vi "LC1_Comm_main.vi"() -> ()   [LabVIEW 2016]
uses:
  <vilib>/DNP3/DNP3_Master/Operation Mode.ctl
  <vilib>/DNP3/DNP3_Master/Poll Binary Input Variation.ctl
  <vilib>/DNP3/DNP3_Master/Analog Variation.ctl
  <vilib>/DNP3/DNP3_Master/Poll Analog Input Variation.ctl
  <vilib>/DNP3/DNP3_Master/Response Type.ctl
  <vilib>/DNP3/DNP3_Master/Start Stop.ctl
  <vilib>/DNP3/DNP3_Master/Analog Info.ctl
  BESS_LC/LC_BESS_global.vi
  Communication/Global communication.vi
  Communication/Global communication output.vi
  Communication/DNP3 communication files/MGCC Communication Files/DNP3_Master_Station_MGCC.lvlib
  <vilib>/DNP3/DNP3_Master.lvlib
panel:
  out "Startup time":dbl
  out "Array":T3(array[cluster])=[{"DNP3 channel"="Master/Channel 160.36.56.202: 18000", "DNP3 master"="Master", "DNP3 master session"="Master/Channel 160.36.56.202: 18000/Master Session 7-8", "DNP3 command"="Master/Channel 160.36.56.202: 18000/Master Session 7-8/Command ", "MS_Network_Settings_Initial"={"Outstation IP"="160.36.56.202", "DNP3 Port"=18000, "DNP3 Master Address"=7, "DNP3 Outstation Address"=8}, "Ping status"=enum."Success", "PollD"=[{"start"=0, "stop"=5}], "PollA"=[{"start"=0, "stop"=5}], "error out"={"status"=FALSE, "code"=5103, "source"="DNP3_Master_Station_MGCC.lvlib:LC1_MS_Main.vi:580001<ERR>\nCommunication timeout\n\n\n<b>Complete call chain:</b>\n     DNP3_Master_Station_MGCC.lvlib:LC1_MS_Main.vi:580001\n     LC1_Comm_main.vi"}, "MS_RESET_IND"=FALSE}, {"DNP3 channel"="Master #1/Channel 160.36.56.201: 18000", "DNP3 master"="Master #1", "DNP3 master session"="Master #1/Channel 160.36.56.201: 18000/Master Session 5-6", "DNP3 command"="Master #1/Channel 160.36.56.201: 18000/Master Session 5-6/Command ", "MS_Network_Settings_Initial"={"Outstation IP"="160.36.56.201", "DNP3 Port"=18000, "DNP3 Master Address"=5, "DNP3 Outstation Address"=6}, "Ping status"=enum."Success", "PollD"=[{"start"=0, "stop"=5}], "PollA"=[{"start"=0, "stop"=5}], "error out"={"status"=FALSE, "code"=5103, "source"="DNP3_Master_Station_MGCC.lvlib:LC1_MS_Main.vi:580001<ERR>\nCommunication timeout\n\n\n<b>Complete call chain:</b>\n     DNP3_Master_Station_MGCC.lvlib:LC1_MS_Main.vi:580001\n     LC1_Comm_main.vi"}, "MS_RESET_IND"=FALSE}, {"DNP3 channel"="Master #2/Channel 160.36.56.208: 18000", "DNP3 master"="Master #2", "DNP3 master session"="Master #2/Channel 160.36.56.208: 18000/Master Session 11-12", "DNP3 command"="Master #2/Channel 160.36.56.208: 18000/Master Session 11-12/Command ", "MS_Network_Settings_Initial"={"Outstation IP"="160.36.56.208", "DNP3 Port"=18000, "DNP3 Master Address"=11, "DNP3 Outstation Address"=12}, "Ping status"=enum."Success", "PollD"=[{"start"=0, "stop"=5}], "PollA"=[{"start"=0, "stop"=5}], "error out"={"status"=FALSE, "code"=5103, "source"="DNP3_Master_Station_MGCC.lvlib:LC1_MS_Main.vi:580001<ERR>\nCommunication timeout\n\n\n<b>Complete call chain:</b>\n     DNP3_Master_Station_MGCC.lvlib:LC1_MS_Main.vi:580001\n     LC1_Comm_main.vi"}, "MS_RESET_IND"=FALSE}]
  out "BESS LC communication":dbl[](array[numeric])=[1.0, 0.9550008993297726, 89.78142055267412, -10.000000000000082, -1.796889843993238, 0.5]
  out "millisecond timer value":u32=199
  in  "LC1_MS_Network_Settings 3":T4={"Outstation IP"="160.36.56.208", "DNP3 Port"=18000, "DNP3 Master Address"=11, "DNP3 Outstation Address"=12}
  in  "Poll Enable 3":T5={"En_Rx_An"=TRUE, "En_Tx_An"=TRUE, "En_Rx_Di"=FALSE, "En_Tx_Di"=FALSE}
  in  "ENABLE MS 3":bool=TRUE
  in  "RESET MS 3":bool caption="Reset Outstation"
  in  "LC1_MS_DNP3_Settings 3":T10={"Binary Out Mode"=6, "Binary In Variation"=0, "Analog Out Variation"=4, "Analog Out Mode"=6, "Analog In Variation"=6} {"Analog In Variation" items=["Default", "32-bit with Flag", "16-bit with Flag", "32-bit without Flag", "16-bit without Flag", "Single-prec with Flag", "Double-prec with Flag"]; "Analog Out Mode" items=["SBO"=0, "Select"=3, "Operate"=4, "Direct"=5, "Direct No Ack"=6]; "Analog Out Variation" items=["32-bit"=1, "16-bit"=2, "Single-prec"=3, "Double-prec"=4]; "Binary In Variation" items=["Default", "Packed Format", "With Flags"]; "Binary Out Mode" items=["SBO"=0, "Select"=3, "Operate"=4, "Direct"=5, "Direct No Ack"=6]}
  out "OS SubVI Iterations":i16=6914
  in  "RESET OS":bool caption="Reset Outstation"
  in  "ENABLE OS":bool=TRUE
  out "OS SETTINGS CHANGED":bool
  out "MS POLLING? IND":bool=TRUE
  in  "Settings Cluster":T11={"Default Variation:Analog Input Event (OBJ32)"=1, "Default Variation:Analog Input (OBJ30)"=1, "Default Variation:Binary Input (OBJ01)"=1, "Default Variation:Analog Output (OBJ40)"=4, "Default Variation:Binary Output Event (OBJ11)"=1, "Default Variation:Binary Output (OBJ10)"=1, "Default Variation:Analog Output Event (OBJ42)"=8, "Unsolicited Response Allowed"=FALSE, "Control:Select Timeout (ms)"=0, "Misc:Appl Confirmation Timeout"=0} {"Default Variation:Analog Output Event (OBJ42)" items=["32-bit without Time"=1, "16-bit without Time"=2, "32-bit with Time"=3, "16-bit with Time"=4, "Single-prec without Time"=5, "Double-prec without Time"=6, "Single-prec with Time"=7, "Double-prec with Time"=8]; "Default Variation:Binary Output (OBJ10)" items=["Packed Format"=1, "Output Status with Flags"=2]; "Default Variation:Binary Output Event (OBJ11)" items=["Status without Time"=1, "Status with Time"=2]; "Default Variation:Analog Output (OBJ40)" items=["32-bit with Flag"=1, "16-bit with Flag"=2, "Single-prec with Flag"=3, "Double-prec with Flag"=4]; "Default Variation:Binary Input (OBJ01)" items=["Packed Format"=1, "With Flags"=2]; "Default Variation:Analog Input (OBJ30)" items=["32-bit with Flag"=1, "16-bit with Flag"=2, "32-bit without Flag"=3, "16-bit without Flag"=4, "Single-prec with Flag"=5, "Double-prec with Flag"=6]; "Default Variation:Analog Input Event (OBJ32)" items=["32-bit without Time"=1, "16-bit without Time"=2, "32-bit with Time"=3, "16-bit with Time"=4, "Single-prec without Time"=5, "Double-prec without Time"=6, "Single-prec with Time"=7, "Double-prec with Time"=8]}
  in  "Network Settings 1":T12={"port (20000)"=18000, "Master IP"="10.38.59.110", "Master Address"=12345, "Outstation Address "=54321, " update rate"=50}
  in  "DNP3 DataMap 1":T13={"Binary Output Points"=1, "Binary Input Points"=0, "Analog Output Points"=62, "Analog Input Points"=62}
  out "Numeric 3":i32
  out "LC1_MS_TX_Status_Binary":T1=enum."Cancel"
  out "LC1_MS_TX_Status_Analog":T1=enum."Success"
  out "LC1_MS_RX_Status_Binary":T1=enum."Cancel"
  out "LC1_MS_RX_Status_Analog":T1=enum."Success"
  out "Analog Input":dbl[](array[numeric])=[1.0, 0.9550008993297726, 89.78142055267412, -10.000000000000082, -1.796889843993238, 0.5]
  in  "LC1_MS_Network_Settings":T4={"Outstation IP"="160.36.56.202", "DNP3 Port"=18000, "DNP3 Master Address"=7, "DNP3 Outstation Address"=8}
  in  "LC1_MS_Network_Settings 2":T4={"Outstation IP"="160.36.56.201", "DNP3 Port"=18000, "DNP3 Master Address"=5, "DNP3 Outstation Address"=6}
  in  "Poll Enable":T5={"En_Rx_An"=TRUE, "En_Tx_An"=TRUE, "En_Rx_Di"=FALSE, "En_Tx_Di"=FALSE}
  in  "Poll Enable 2":T5={"En_Rx_An"=TRUE, "En_Tx_An"=TRUE, "En_Rx_Di"=FALSE, "En_Tx_Di"=FALSE}
  in  "ENABLE MS":bool=TRUE
  in  "ENABLE MS 2":bool=TRUE
  in  "RESET MS 2":bool caption="Reset Outstation"
  in  "RESET MS":bool caption="Reset Outstation"
  in  "LC1_MS_DNP3_Settings":T10={"Binary Out Mode"=6, "Binary In Variation"=0, "Analog Out Variation"=4, "Analog Out Mode"=6, "Analog In Variation"=6} {"Analog In Variation" items=["Default", "32-bit with Flag", "16-bit with Flag", "32-bit without Flag", "16-bit without Flag", "Single-prec with Flag", "Double-prec with Flag"]; "Analog Out Mode" items=["SBO"=0, "Select"=3, "Operate"=4, "Direct"=5, "Direct No Ack"=6]; "Analog Out Variation" items=["32-bit"=1, "16-bit"=2, "Single-prec"=3, "Double-prec"=4]; "Binary In Variation" items=["Default", "Packed Format", "With Flags"]; "Binary Out Mode" items=["SBO"=0, "Select"=3, "Operate"=4, "Direct"=5, "Direct No Ack"=6]}
  in  "LC1_MS_DNP3_Settings 2":T10={"Binary Out Mode"=6, "Binary In Variation"=0, "Analog Out Variation"=4, "Analog Out Mode"=6, "Analog In Variation"=6} {"Analog In Variation" items=["Default", "32-bit with Flag", "16-bit with Flag", "32-bit without Flag", "16-bit without Flag", "Single-prec with Flag", "Double-prec with Flag"]; "Analog Out Mode" items=["SBO"=0, "Select"=3, "Operate"=4, "Direct"=5, "Direct No Ack"=6]; "Analog Out Variation" items=["32-bit"=1, "16-bit"=2, "Single-prec"=3, "Double-prec"=4]; "Binary In Variation" items=["Default", "Packed Format", "With Flags"]; "Binary Out Mode" items=["SBO"=0, "Select"=3, "Operate"=4, "Direct"=5, "Direct No Ack"=6]}
  out "Number of iteration":i32=3464
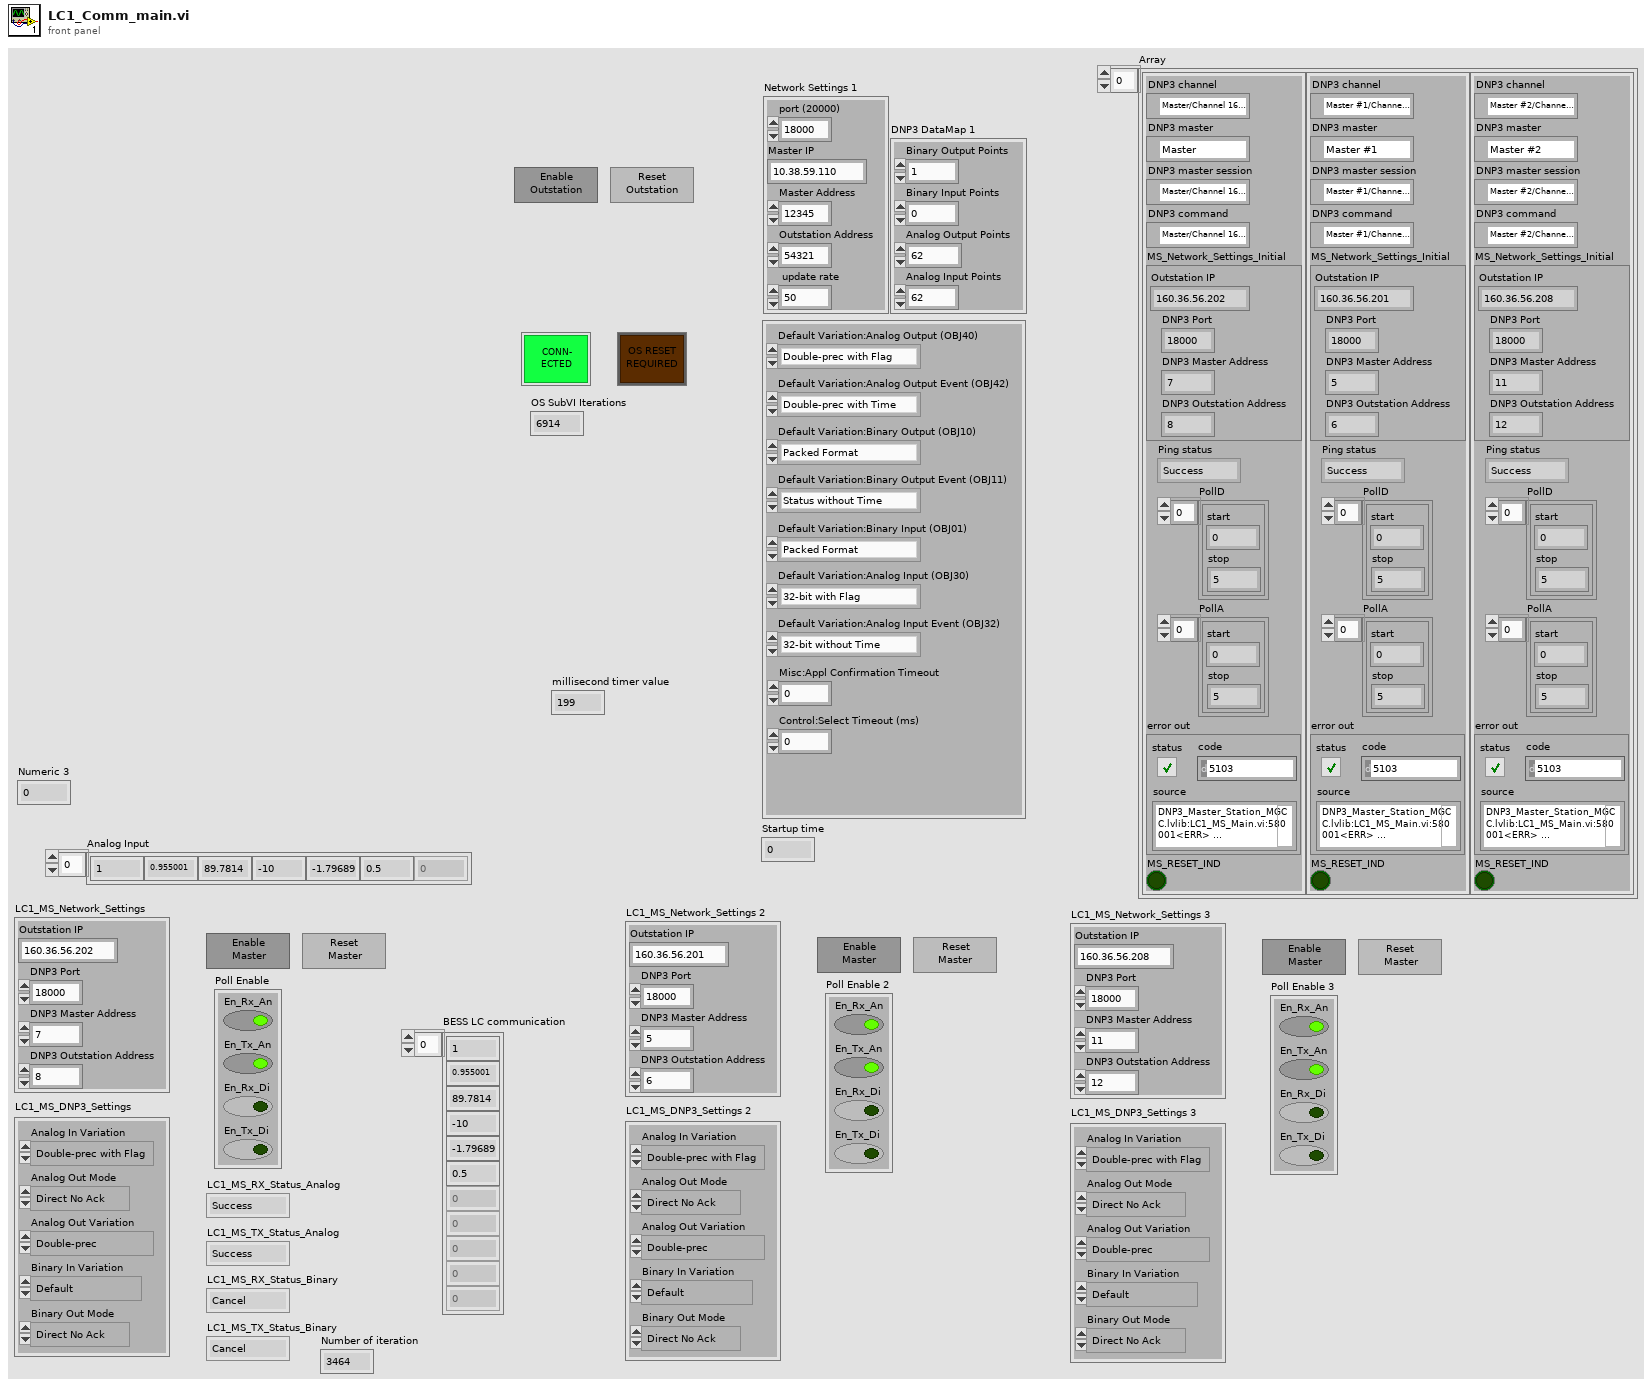
[diagram p1: front panel]
types:
  T1 = typedef "DNP3_Master.lvlib/Response Type.ctl" = enum16{"Idle", "Buffering", "Pending", "Success", "Failure", "Mismatch", "Status Code", "IIN", "Timeout", "Cancel"}
  T2 = typedef "DNP3_Master.lvlib/Start Stop.ctl" = cluster{"start":u16, "stop":u16}
  T3 = cluster{"DNP3 channel":refnum<k21>, "DNP3 master":refnum<k21>, "DNP3 master session":refnum<k21>, "DNP3 command":refnum<k21>, "MS_Network_Settings_Initial":cluster{"Outstation IP":string, "DNP3 Port":u16, "DNP3 Master Address":u16, "DNP3 Outstation Address":u16}, "Ping status":T1, "PollD":T2[], "PollA":T2[], "error out":errorcluster, "MS_RESET_IND":bool}[]
  T4 = cluster{"Outstation IP":string, "DNP3 Port":u16, "DNP3 Master Address":u16, "DNP3 Outstation Address":u16}
  T5 = cluster{"En_Rx_An":bool, "En_Tx_An":bool, "En_Rx_Di":bool, "En_Tx_Di":bool}
  T6 = typedef "DNP3_Master.lvlib/Operation Mode.ctl" = u8
  T7 = typedef "DNP3_Master.lvlib/Poll Binary Input Variation.ctl" = u8
  T8 = typedef "DNP3_Master.lvlib/Analog Variation.ctl" = u8
  T9 = typedef "DNP3_Master.lvlib/Poll Analog Input Variation.ctl" = u8
  T10 = cluster{"Binary Out Mode":T6, "Binary In Variation":T7, "Analog Out Variation":T8, "Analog Out Mode":T6, "Analog In Variation":T9}
  T11 = cluster{"Default Variation:Analog Input Event (OBJ32)":u8, "Default Variation:Analog Input (OBJ30)":u8, "Default Variation:Binary Input (OBJ01)":u8, "Default Variation:Analog Output (OBJ40)":u8, "Default Variation:Binary Output Event (OBJ11)":u8, "Default Variation:Binary Output (OBJ10)":u8, "Default Variation:Analog Output Event (OBJ42)":u8, "Unsolicited Response Allowed":bool, "Control:Select Timeout (ms)":u32, "Misc:Appl Confirmation Timeout":u32}
  T12 = cluster{"port (20000)":u16, "Master IP":string, "Master Address":u16, "Outstation Address ":u16, " update rate":u32}
  T13 = cluster{"Binary Output Points":u16, "Binary Input Points":u16, "Analog Output Points":u16, "Analog Input Points":u16}
  T14 = typedef "DNP3_Master.lvlib/Analog Info.ctl" = cluster{"index":u16, "value":dbl}
  T15 = cluster{"Binary Out Mode":T6, "Binary In Variation":T7, "Analog Out Variation":T8, "Analog Out Mode":T6, "Analog In Variation":T9}[]
  T16 = cluster{"En_Rx_An":bool, "En_Tx_An":bool, "En_Rx_Di":bool, "En_Tx_Di":bool}[]
  T17 = cluster{"Outstation IP":string, "DNP3 Port":u16, "DNP3 Master Address":u16, "DNP3 Outstation Address":u16}[]
  T18 = cluster{"response status":T1, "response status":T1, "response status":T1, "response status":T1}
  T19 = cluster{"DNP3 channel":refnum<k21>, "DNP3 master":refnum<k21>, "DNP3 master session":refnum<k21>, "DNP3 command":refnum<k21>, "MS_Network_Settings_Initial":cluster{"Outstation IP":string, "DNP3 Port":u16, "DNP3 Master Address":u16, "DNP3 Outstation Address":u16}, "Ping status":T1, "PollD":T2[], "PollA":T2[], "error out":errorcluster, "MS_RESET_IND":bool}
  T20 = cluster{"DNP3 outstation session out":refnum<k21>, "DNP3 outstation out":refnum<k21>, "error out":errorcluster}
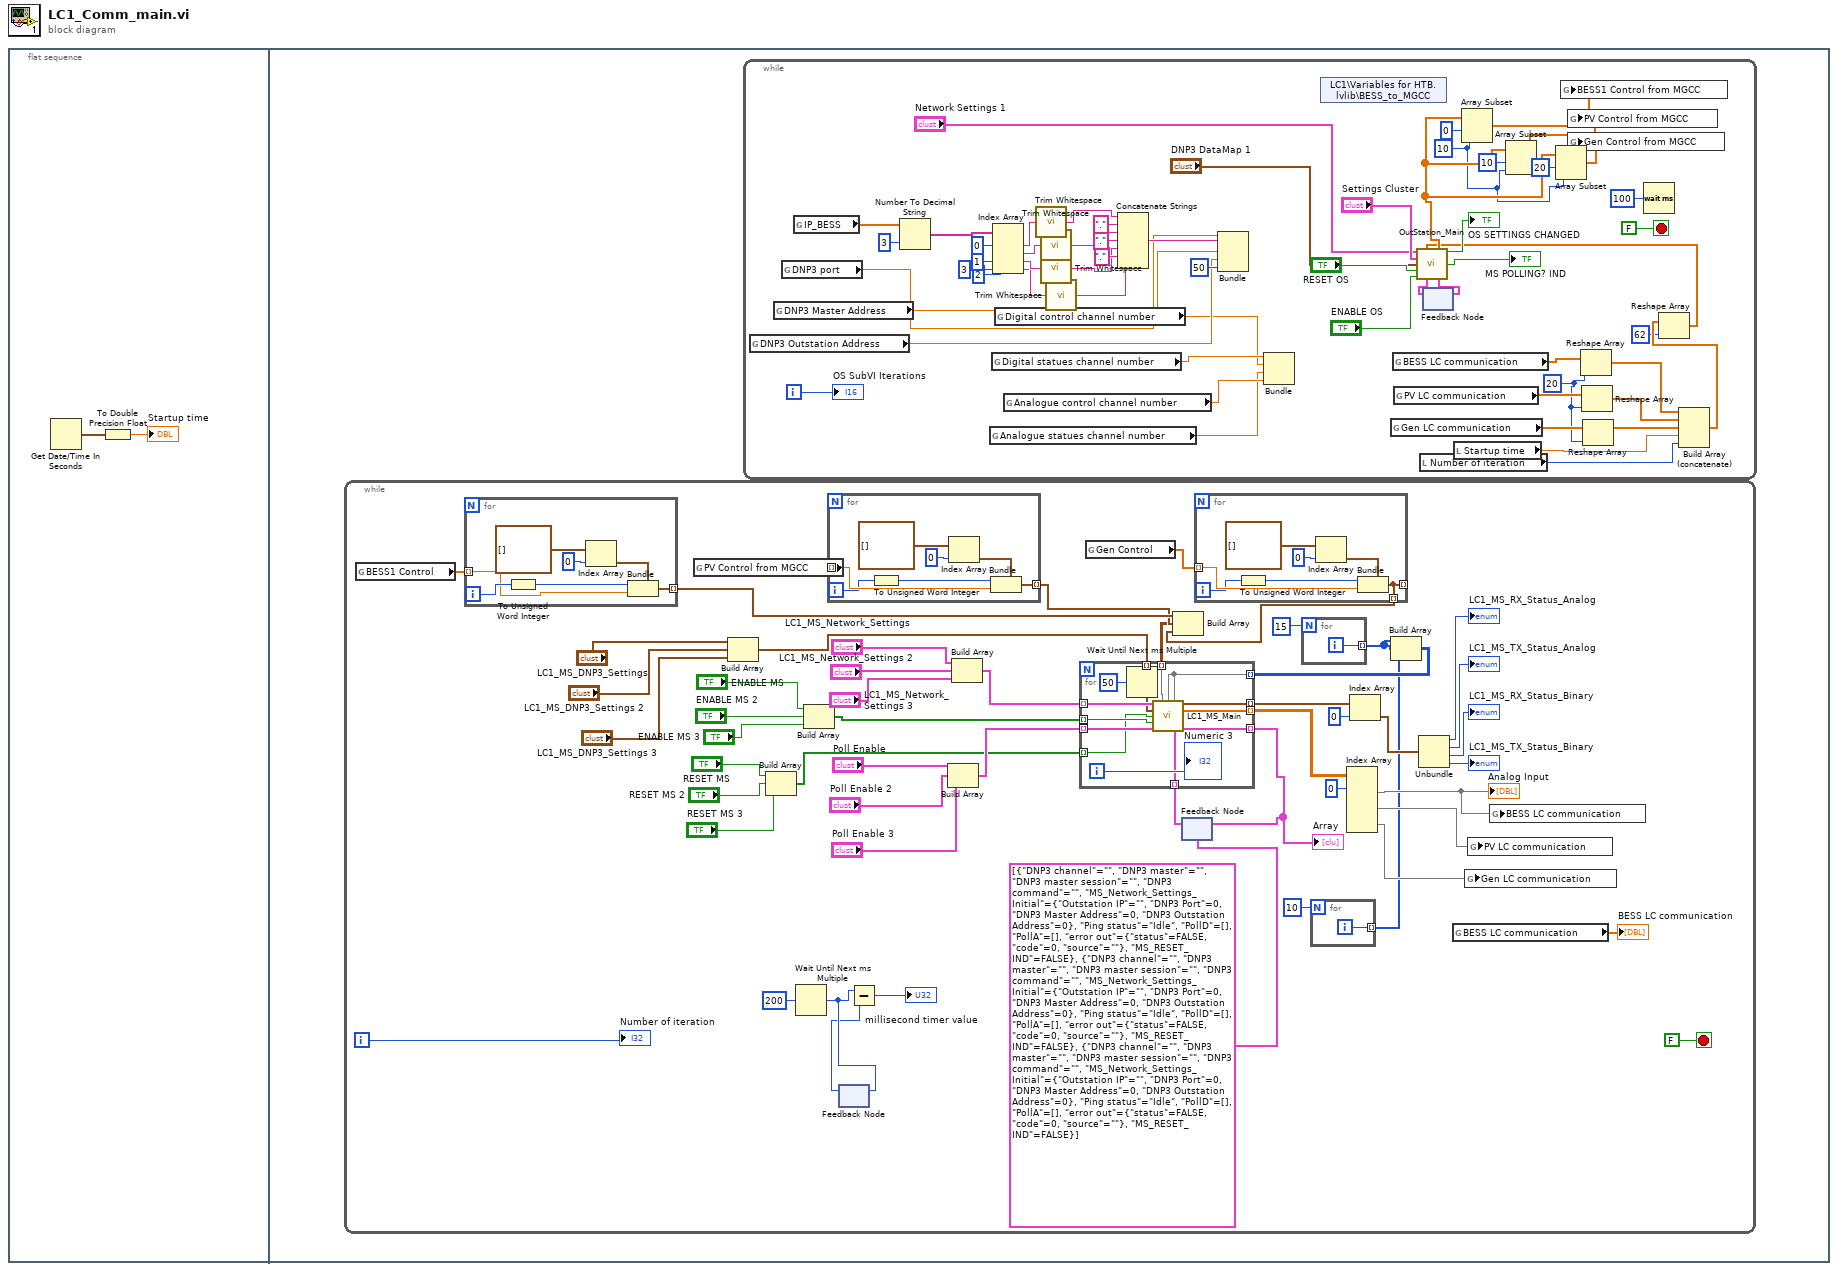
[diagram p0: block diagram]
diagram:
  n1 = flat-sequence {
    frame #0 {
      n2 = Get Date/Time In Seconds() -> (seconds since 1Jan1904=w2:timestamp)
      n3 = To Double Precision Float(number=w2) -> (double precision float=→"Startup time":dbl)
    }
    frame #1 {
      n4 = while {
        i -> [w25]
        stop <- FALSE stop-if-true
        n5 = global read "Global communication output.vi" "BESS1 Control"() -> (w30:dbl[])
        n6 = for {
          tunnel: [w79] -> w28 mode=indexing
          tunnel: w30 -> [w73] mode=indexing
          i -> [w74]
          n7 = To Unsigned Word Integer(number=w74) -> (unsigned 16bit integer=w75:u16)
          n8 = Index Array(array=T14[] [] ("values"), index=0) -> (element=w76:T14)
          n9 = Bundle(cluster=w76, "index"=w75, "value"=w73) -> (w79:T14)
        }
        n10 = global read "Global communication output.vi" "PV Control from MGCC"() -> (w29:dbl[])
        n11 = Build Array("LC1_MS_DNP3_Settings", "LC1_MS_DNP3_Settings 2", "LC1_MS_DNP3_Settings 3") -> (w31:T15)
        n12 = Build Array("RESET MS", "RESET MS 2", "RESET MS 3") -> (w34:bool[])
        n13 = Wait Until Next ms Multiple(millisecond multiple=u32 200) -> (millisecond timer value=w15:u32)
        n14 = Build Array("ENABLE MS", "ENABLE MS 2", "ENABLE MS 3") -> (w37:bool[])
        n15 = for {
          tunnel: [w72] -> w27 mode=indexing
          tunnel: w29 -> [w67] mode=indexing
          i -> [w66]
          n16 = To Unsigned Word Integer(number=w66) -> (unsigned 16bit integer=w68:u16)
          n17 = Index Array(array=T14[] [] ("values"), index=0) -> (element=w69:T14)
          n18 = Bundle(cluster=w69, "index"=w68, "value"=w67) -> (w72:T14)
        }
        n19 = feedback-in #1(w15) -> ()
        n20 = feedback #1() -> (w14:u32)  [unwired: 1 in]
        n21 = Subtract(x=w15, y=w14) -> (x-y=→"millisecond timer value":u32)
        n22 = Build Array("Poll Enable", "Poll Enable 2", "Poll Enable 3") -> (w40:T16)
        n23 = Build Array("LC1_MS_Network_Settings", "LC1_MS_Network_Settings 2", "LC1_MS_Network_Settings 3") -> (w43:T17)
        n24 = global read "Global communication output.vi" "Gen Control"() -> (w3:dbl[])
        n25 = feedback #2(T3 [{"DNP3 channel"="", "DNP3 master"="", "DNP3 master session"="", "DNP3 command"="", "MS_Network_Settings_Initial"={"Outstation IP"="", "DNP3 Port"=0, "DNP3 Master Address"=0, "DNP3 Outstation Address"=0}, "Ping status"=enum."Idle", "PollD"=[], "PollA"=[], "error out"={"status"=FALSE, "code"=0, "source"=""}, "MS_RESET_IND"=FALSE}, {"DNP3 channel"="", "DNP3 master"="", "DNP3 master session"="", "DNP3 command"="", "MS_Network_Settings_Initial"={"Outstation IP"="", "DNP3 Port"=0, "DNP3 Master Address"=0, "DNP3 Outstation Address"=0}, "Ping status"=enum."Idle", "PollD"=[], "PollA"=[], "error out"={"status"=FALSE, "code"=0, "source"=""}, "MS_RESET_IND"=FALSE}, {"DNP3 channel"="", "DNP3 master"="", "DNP3 master session"="", "DNP3 command"="", "MS_Network_Settings_Initial"={"Outstation IP"="", "DNP3 Port"=0, "DNP3 Master Address"=0, "DNP3 Outstation Address"=0}, "Ping status"=enum."Idle", "PollD"=[], "PollA"=[], "error out"={"status"=FALSE, "code"=0, "source"=""}, "MS_RESET_IND"=FALSE}]) -> (w22:T3)
        n26 = for {
          tunnel: [w59] -> _ mode=indexing
          tunnel: w3 -> [w61] mode=indexing
          tunnel: [w59] -> w16 mode=indexing
          i -> [w60]
          n27 = To Unsigned Word Integer(number=w60) -> (unsigned 16bit integer=w62:u16)
          n28 = Index Array(array=T14[] [] ("values"), index=0) -> (element=w63:T14)
          n29 = Bundle(cluster=w63, "index"=w62, "value"=w61) -> (w59:T14)
        }
        n30 = Build Array(w28, w27, w16) -> (w26:T14[][])
        n31 = for {
          N: 15 -> [_]
          tunnel: [w58] -> w7 mode=indexing
          i -> [w58]
        }
        n32 = for {
          N: 10 -> [_]
          tunnel: [w57] -> w5 mode=indexing
          i -> [w57]
        }
        n33 = Build Array(w7, w7, w5) -> (w6:i32[][])
        n34 = for {
          tunnel: [w92] -> w52 mode=indexing
          tunnel: [w91] -> w47 mode=indexing
          tunnel: w43 -> [w90] mode=indexing
          tunnel: [w89] -> w23 mode=indexing
          tunnel: w40 -> [w88] mode=indexing
          tunnel: w37 -> [w87] mode=indexing
          tunnel: w34 -> [w86] mode=indexing
          tunnel: w31 -> [w85] mode=indexing
          tunnel: w26 -> [w84] mode=indexing
          tunnel: w6 -> [w83] mode=indexing
          tunnel: w22 -> [w80] mode=indexing
          i -> [w82]
          n35 = Wait Until Next ms Multiple(millisecond multiple=u32 50) -> ()  [unwired: 1 out]
          n36 = call "LC1_MS_Main.vi"("MS_Network_Settings"=w90, "Analog Output"=w84, "Analog Input Indexes"=w83, "Digital Input Indexes"=w83, "MS_DNP3_Settings"=w85, "MS_RESET"=w86, "MS_ENABLE"=w87, "Poll Enable"=w88, "DNP3 Session Feedback"=w80) -> ("Comm Status"=w92:T18, "Analog Input"=w91:dbl[], "DNP3 Session Output"=w89:T19)  [unwired: 3 in, 1 out]
          "Numeric 3" <- w82
        }
        "Array" <- w23
        n37 = feedback-in #2(w23) -> ()
        n38 = Index Array(array=w47, index (row) #1=0 ("index")) -> (element #1=w48:dbl[], element #2=w10:dbl[], element #3=w9:dbl[])  [unwired: 5 in]
        "Analog Input" <- w48
        n39 = Index Array(array=w52, index=0) -> (element=w51:T18)
        n40 = Unbundle(w51) -> ("response status"=→"LC1_MS_RX_Status_Analog":T1, "response status"=→"LC1_MS_TX_Status_Analog":T1, "response status"=→"LC1_MS_RX_Status_Binary":T1, "response status"=→"LC1_MS_TX_Status_Binary":T1)
        n41 = global read "Global communication.vi" "BESS LC communication"() -> (→"BESS LC communication":dbl[])
        n42 = global write "Global communication.vi" "Gen LC communication"(w9) -> ()
        n43 = global write "Global communication.vi" "PV LC communication"(w10) -> ()
        n44 = global write "Global communication.vi" "BESS LC communication"(w48) -> ()
        "Number of iteration" <- w25
      }
      n45 = while {
        i -> [w149]
        stop <- FALSE stop-if-true
        w108 = 10 ("length")
        w98 = 20 ("dimension size")
        n46 = global read "LC_BESS_global.vi" "DNP3 Outstation Address"() -> (w126:dbl)
        n47 = global read "LC_BESS_global.vi" "DNP3 Master Address"() -> (w127:dbl)
        n48 = global read "LC_BESS_global.vi" "DNP3 port"() -> (w128:dbl)
        n49 = global read "LC_BESS_global.vi" "IP_BESS"() -> (w147:dbl[])
        n50 = Number To Decimal String(number=w147, width (-)=i16 3) -> (decimal integer string=w145:string[])
        n51 = global read "LC_BESS_global.vi" "Analogue statues channel number"() -> (w122:dbl)
        n52 = global read "LC_BESS_global.vi" "Digital statues channel number"() -> (w125:dbl)
        n53 = Index Array(array=w145, index #1=0 ("index"), index #2=1 ("index"), index #3=2 ("index"), index #4=3 ("index")) -> (element #1=w137:string, element #2=w135:string, element #3=w133:string, element #4=w131:string)
        n54 = global read "LC_BESS_global.vi" "Digital control channel number"() -> (w124:dbl)
        n55 = global read "LC_BESS_global.vi" "Analogue control channel number"() -> (w123:dbl)
        n56 = call <vilib>:"Trim Whitespace.vi"("string"=w137) -> ("trimmed string"=w136:string)  [unwired: 1 in]
        n57 = call <vilib>:"Trim Whitespace.vi"("string"=w135) -> ("trimmed string"=w134:string)  [unwired: 1 in]
        n58 = call <vilib>:"Trim Whitespace.vi"("string"=w133) -> ("trimmed string"=w132:string)  [unwired: 1 in]
        n59 = call <vilib>:"Trim Whitespace.vi"("string"=w131) -> ("trimmed string"=w130:string)  [unwired: 1 in]
        n60 = Concatenate Strings(w136, "." ("string"), w134, "." ("string"), w132, "." ("string"), w130) -> (w129:string)
        n61 = Bundle("DNP3 port"=w128, w129, "DNP3 Master Address"=w127, "DNP3 Outstation Address"=w126, "update rate"=u32 50) -> ()  [unwired: 1 in, 1 out]
        n62 = Bundle("Digital statues channel number"=w125, "Digital control channel number"=w124, "Analogue statues channel number"=w122, "Analogue control channel number"=w123) -> ()  [unwired: 1 in, 1 out]
        n63 = shared-variable "LC1\\Variables for HTB.lvlib\\BESS_to_MGCC"() -> ()  [unwired: 1 in, 2 out]
        n64 = global read "Global communication.vi" "Gen LC communication"() -> (w99:dbl[])
        n65 = global read "Global communication.vi" "BESS LC communication"() -> (w104:dbl[])
        n66 = global read "Global communication.vi" "PV LC communication"() -> (w100:dbl[])
        n67 = local read "Number of iteration"() -> (w93:i32)
        n68 = feedback #3() -> (w117:T20)  [unwired: 1 in]
        n69 = local read "Startup time"() -> (w94:dbl)
        n70 = Reshape Array(w104, w98) -> (w103:dbl[])
        n71 = Reshape Array(w100, w98) -> (w102:dbl[])
        n72 = Reshape Array(w99, w98) -> (w101:dbl[])
        n73 = Wait (ms)(milliseconds to wait=u32 100) -> ()  [unwired: 1 out]
        n74 = Build Array (concatenate)(w103, w102, w101, w94, w93) -> (w97:dbl[])
        n75 = Reshape Array(w97, 62 ("dimension size")) -> (w95:dbl[])
        n76 = call "OutStation_Main.vi"("Network Settings 1"="Network Settings 1", "Analog Input"=w95, "Settings Cluster"="Settings Cluster", "DNP3 DataMap 1"="DNP3 DataMap 1", "OS_Reset"="RESET OS", "OS_Enable"="ENABLE OS", "DNP3 Session Input"=w117) -> ("Analog Output"=w109:dbl[], "OS_DNP3_Settings_Changed"=→"OS SETTINGS CHANGED":bool, "Connected?"=→"MS POLLING? IND":bool, "DNP3 Session"=w118:T20)  [unwired: 2 in, 3 out]
        n77 = feedback-in #3(w118) -> ()
        n78 = Array Subset(array=w109, index=0, length=w108) -> (w112:dbl[])
        n79 = Array Subset(array=w109, index=10, length=w108) -> (w106:dbl[])
        n80 = Array Subset(array=w109, index=20, length=w108) -> (w105:dbl[])
        n81 = global write "Global communication output.vi" "BESS1 Control from MGCC"(w112) -> ()
        n82 = global write "Global communication output.vi" "PV Control from MGCC"(w106) -> ()
        n83 = global write "Global communication output.vi" "Gen Control from MGCC"(w105) -> ()
        "OS SubVI Iterations" <- w149
      }
    }
  }
